vi "Previous Element Sum.vi"() -> ()   [LabVIEW 2024]
panel:
  out "Output array":dbl[](array[numeric])
  in  "Input array":dbl[](array[numeric])
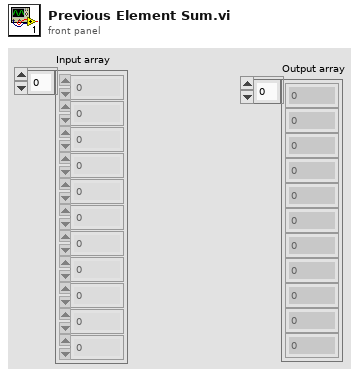
[diagram p1: front panel]
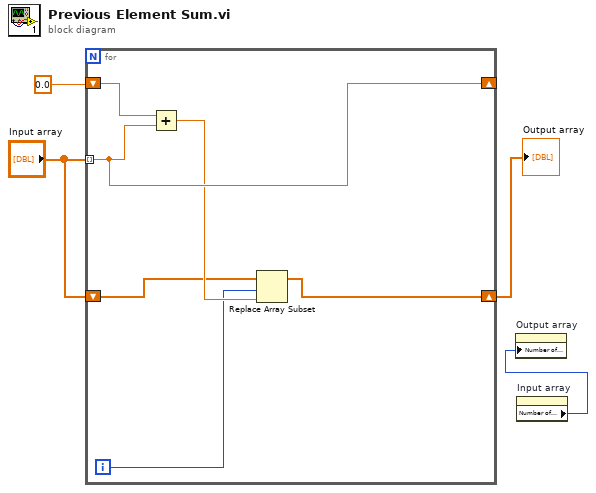
[diagram p0: block diagram]
diagram:
  n1 = for {
    tunnel: "Input array" -> [w9] mode=indexing
    shift-right: [w5] -> w2
    shift-left: "Input array" -> [w6]
    shift-right: [w9] -> _
    shift-left: 0.0 -> [w10]
    i -> [w7]
    n2 = Add(x=w10, y=w9) -> (x+y=w8:dbl)
    n3 = Replace Array Subset(array=w6, new element=w8, index=w7) -> (w5:dbl[])
  }
  "Output array" <- w2
  n4 = property on="Input array" class="Arr (strict)"() -> ("Number of Rows"=w1:u32)  [unwired: 2 in, 2 out]
  n5 = property on="Output array" class="Arr (strict)"("Number of Rows"=w1) -> ()  [unwired: 2 in, 2 out]
